vi "PC_DDPG to DDPM two lines or ports same DAQ.vi"() -> ()   [LabVIEW 2021]
uses:
  Common/Typedefs/Execution Options - Measure.ctl
  Dynamic Digital Pattern Measurement/Typedefs/Timing & Trigger Settings.ctl
  Dynamic Digital Pattern Measurement/Typedefs/Timing Settings.ctl
  Dynamic Digital Pattern Measurement/Typedefs/Trigger Settings.ctl
  Synchronization/Typedefs/Routing Path.ctl
  Synchronization/Typedefs/Routing Signal.ctl
  Dynamic Digital Pattern Measurement/DAQ_Dynamic Digital Pattern Measurement.lvlib
  Synchronization/DAQ_Synchronization.lvlib
  Dynamic Digital Pattern Generation/DAQ_Dynamic Digital Pattern Generation.lvlib
panel:
  in  "Port Digital Data Out":u32[](array[numeric])=[262144, 615000, 713140, 616421, 679353]
  out "Port Digital Data In":u32[](array[numeric])=[0, 0, 262144, 524288, 262144]
  out "Measured Digital Patterns":digitalwaveform(graph)={"t0"=timestamp(3805346440.5882516 s since 1904-01-01), "dt"=9.999999999999999e-05, "Y"={"transitions"=[], "data"=[[0, 0], [0, 0], [1, 0], [0, 1], [1, 0]]}, "attributes"=variant("NI_ChannelName"=variant(string "Dev1/port0/line18..."), "NI_LineNames"=variant(string "Dev1/port0/line18,Dev1/port0/line19"))}
  out "error out":errorcluster
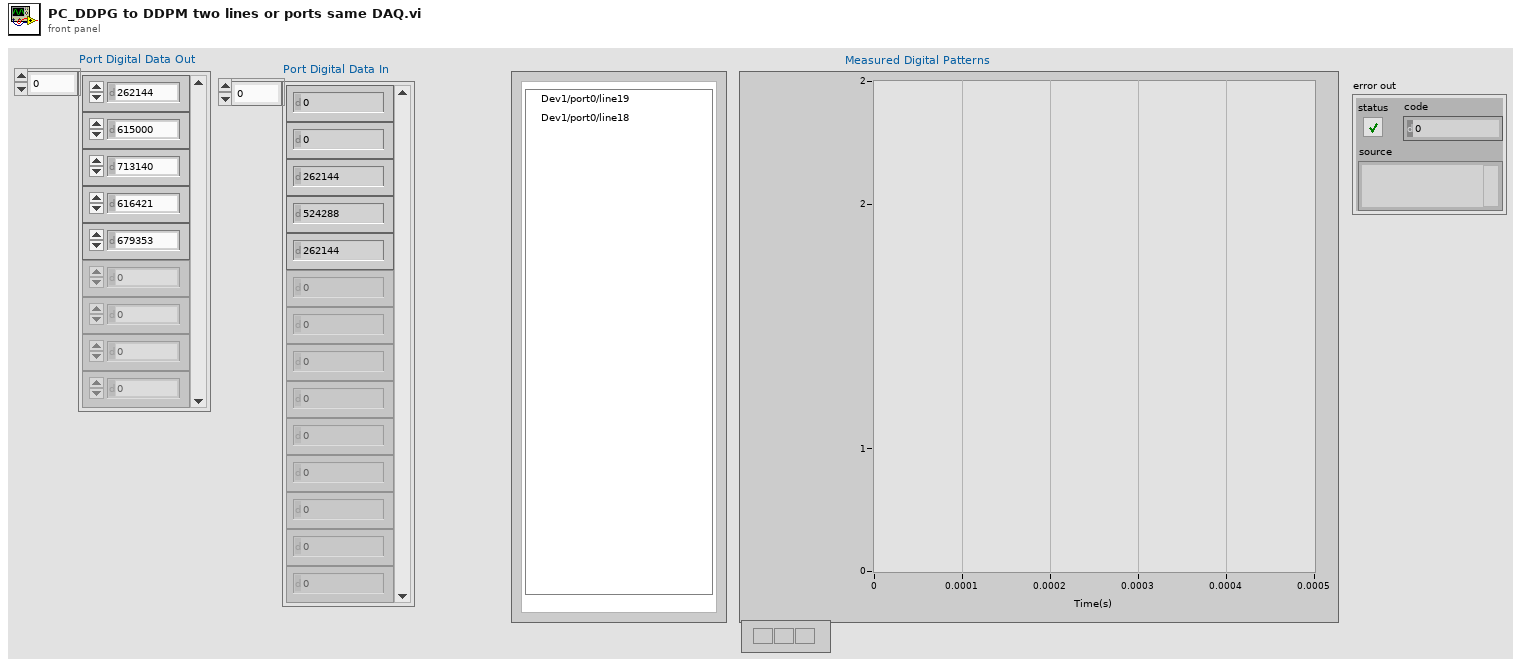
[diagram p1: front panel]
types:
  T1 = typedef "DAQ_Synchronization.lvlib/Routing Path.ctl" = cluster{"Signal":T2, "Output Terminal":tag}
  T2 = typedef "DAQ_Synchronization.lvlib/Routing Signal.ctl" = enum16{"Sample Clock", "Start Trigger"}
  T3 = typedef "DAQ_Dynamic Digital Pattern Measurement.lvlib/Timing & Trigger Settings.ctl" = cluster{"Timing Settings":T4, "Trigger Settings":T5}
  T4 = typedef "DAQ_Dynamic Digital Pattern Measurement.lvlib/Timing Settings.ctl" = cluster{"Sample Clock Source":tag, "Sample Rate (Hz)":dbl, "Number of Samples":i32, "Active Edge":i32}
  T5 = typedef "DAQ_Dynamic Digital Pattern Measurement.lvlib/Trigger Settings.ctl" = cluster{"Trigger Type":enum16{"No Trigger", "Digital Start"}, "Digital Start Trigger Source":tag, "Digital Start Trigger Edge":i32}
  T6 = typedef "Execution Options - Measure.ctl" = enum16{"Configure & Measure", "Configure only", "Measure only"}
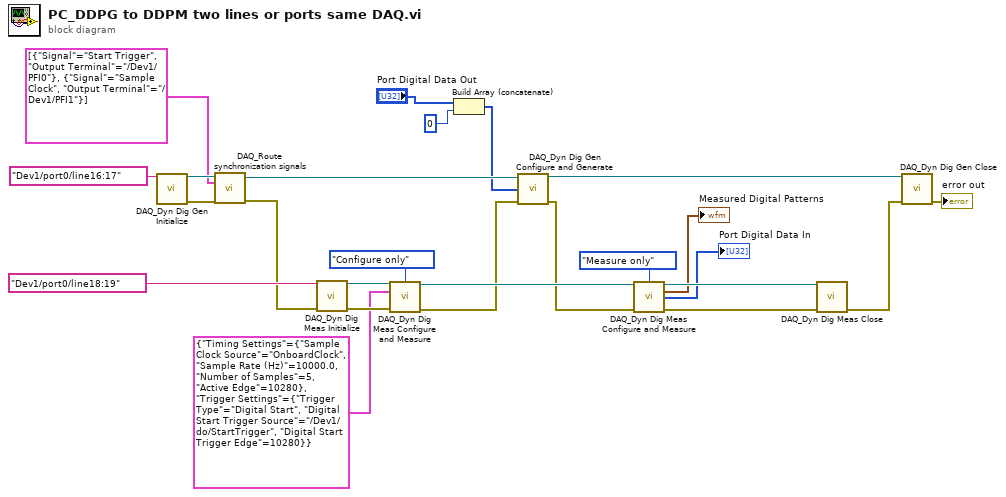
[diagram p0: block diagram]
diagram:
  n1 = call "DAQ_Dyn Dig Gen Initialize.vi"("Physical Channels"=tag "Dev1/port0/line16:17") -> ("DAQmx Task Out"=w9:refnum<k21>, "error out"=w8:errorcluster)  [unwired: 13 in]
  n2 = call "DAQ_Route synchronization signals.vi"("DAQmx Task In"=w9, "Routing paths"=T1[] [{"Signal"=enum."Start Trigger", "Output Terminal"="/Dev1/PFI0"}, {"Signal"=enum."Sample Clock", "Output Terminal"="/Dev1/PFI1"}], "error in"=w8) -> ("DAQmx Task Out"=w6:refnum<k21>, "error out"=w7:errorcluster)  [unwired: 11 in]
  n3 = call "DAQ_Dyn Dig Meas Initialize.vi"("Physical Channels"=tag "Dev1/port0/line18:19", "error in"=w7) -> ("DAQmx Task Out"=w23:refnum<k21>, "error out"=w21:errorcluster)  [unwired: 12 in]
  n4 = call "DAQ_Dyn Dig Meas Configure and Measure.vi"("DAQmx Task In"=w23, "Execution Option"=Execution_Options_-_Measure."Configure only", "Timing and Trigger Settings"=T3 {"Timing Settings"={"Sample Clock Source"="OnboardClock", "Sample Rate (Hz)"=10000.0, "Number of Samples"=5, "Active Edge"=10280}, "Trigger Settings"={"Trigger Type"=enum."Digital Start", "Digital Start Trigger Source"="/Dev1/do/StartTrigger", "Digital Start Trigger Edge"=10280}}, "error in"=w21) -> ("DAQmx Task Out"=w22:refnum<k21>, "error out"=w20:errorcluster)  [unwired: 7 in, 3 out]
  n5 = Build Array (concatenate)("Port Digital Data Out", u32 0 ("new element/subarray")) -> (w2:u32[])
  n6 = call "DAQ_Dyn Dig Gen Configure and Generate.vi"("DAQmx Task In"=w6, "Port Digital Data"=w2, "error in"=w20) -> ("DAQmx Task Out"=w24:refnum<k21>, "error out"=w19:errorcluster)  [unwired: 10 in, 1 out]
  n7 = call "DAQ_Dyn Dig Meas Configure and Measure.vi"("DAQmx Task In"=w22, "Execution Option"=Execution_Options_-_Measure."Measure only", "error in"=w19) -> ("DAQmx Task Out"=w17:refnum<k21>, "Measured Digital Patterns"=→"Measured Digital Patterns":digitalwaveform, "Port Digital Data"=→"Port Digital Data In":u32[], "error out"=w18:errorcluster)  [unwired: 8 in, 1 out]
  n8 = call "DAQ_Dyn Dig Meas Close.vi"("DAQmx Task In"=w17, "error in"=w18) -> ("error out"=w16:errorcluster)  [unwired: 13 in]
  n9 = call "DAQ_Dyn Dig Gen Close.vi"("DAQmx Task In"=w24, "error in"=w16) -> ("error out"=→"error out":errorcluster)  [unwired: 13 in]
